vi "Message Based Application Example.vi"() -> ()   [LabVIEW 2014]
uses:
  <vilib>/Utility/error.llb/DialogType.ctl
  vilib/Message/Msg Post UI Message.vi
  vilib/Message/Msg Post Queue Message.vi
  vilib/Message/Msg Send Queue Message.vi
panel:
  in  "Button 2":bool
  in  "Button 1":bool
  in  "stop":bool
  # "Example buttons to create example events"
  # "Template for a Message Handling Framework-based VI. Add your controls (or menus or whatever) to the front panel here and edit the block diagram to complete the VI. You'll probably also want to delete this label!\n\nCopyright 2005 - 2016 Jason Sommerville\n\nPermision to use, modify and distribute this VI and its subVIs is granted under the BSD license."
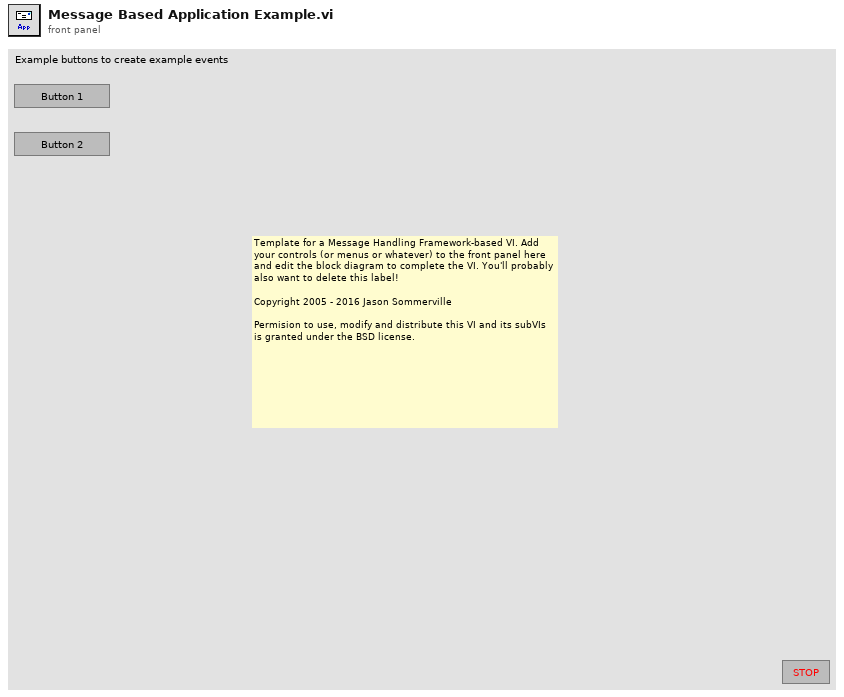
[diagram p1: front panel]
types:
  T1 = typedef "DialogType.ctl" = u16
  T2 = enum16{"Left Button", "Center Button", "Right Button", "Window Close"}
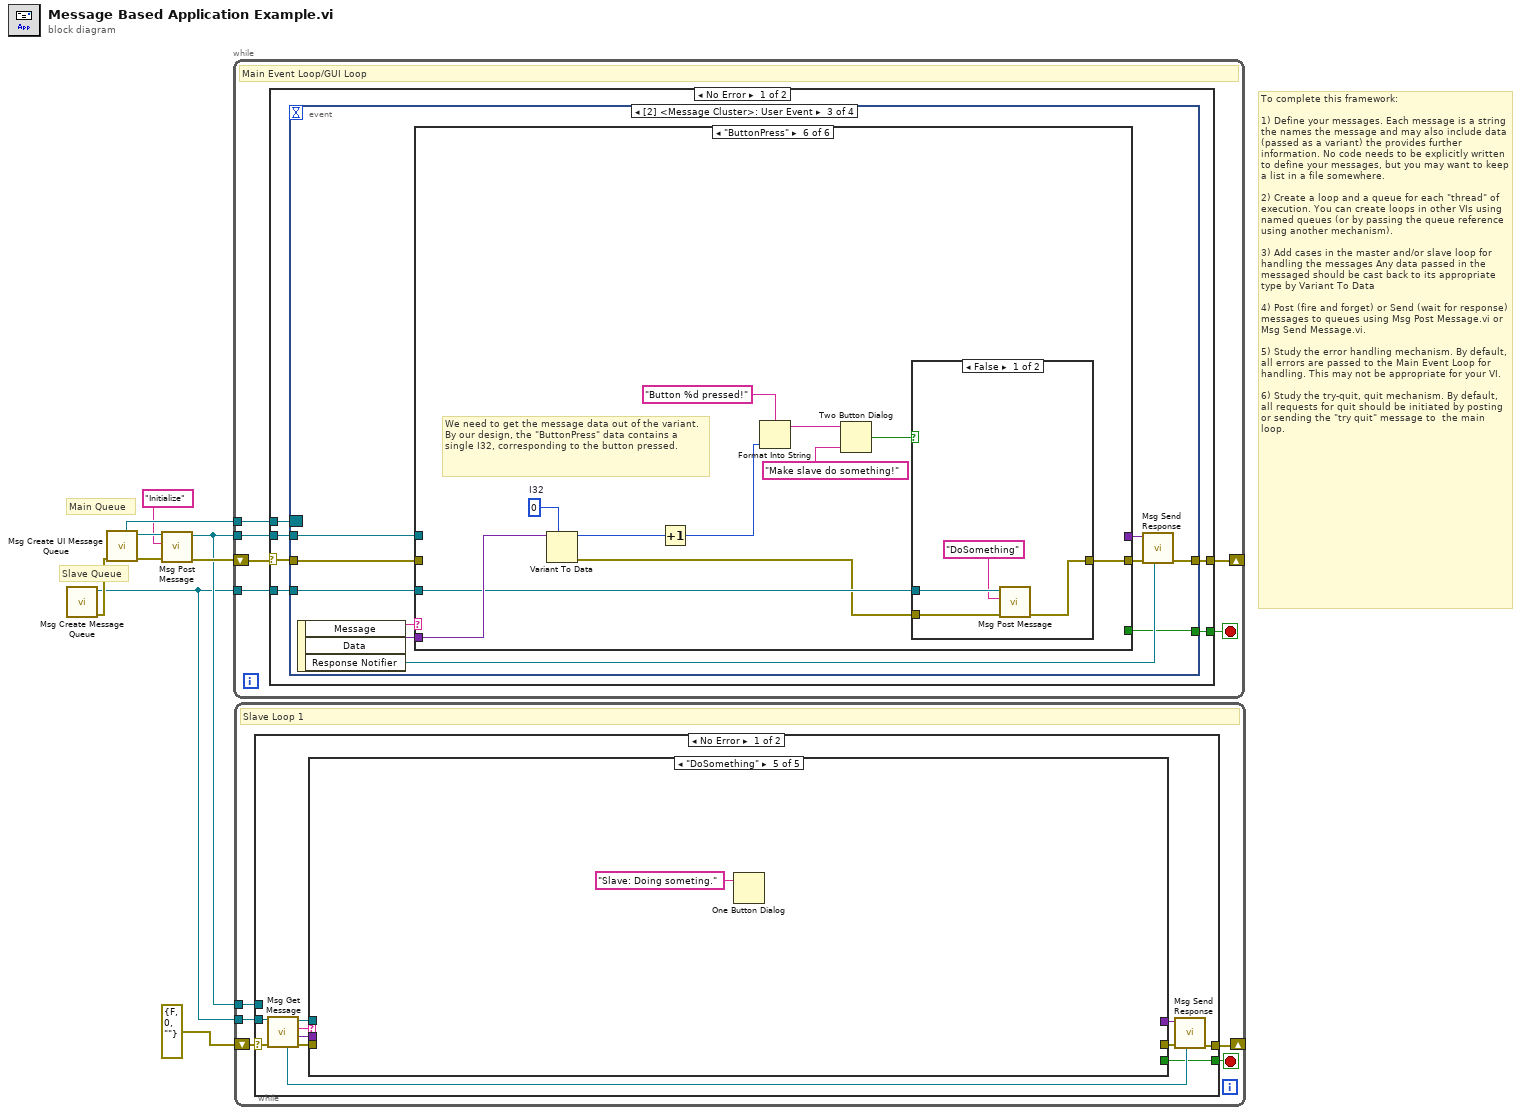
[diagram p0: block diagram]
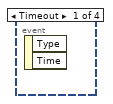
[diagram p2: hidden frame]
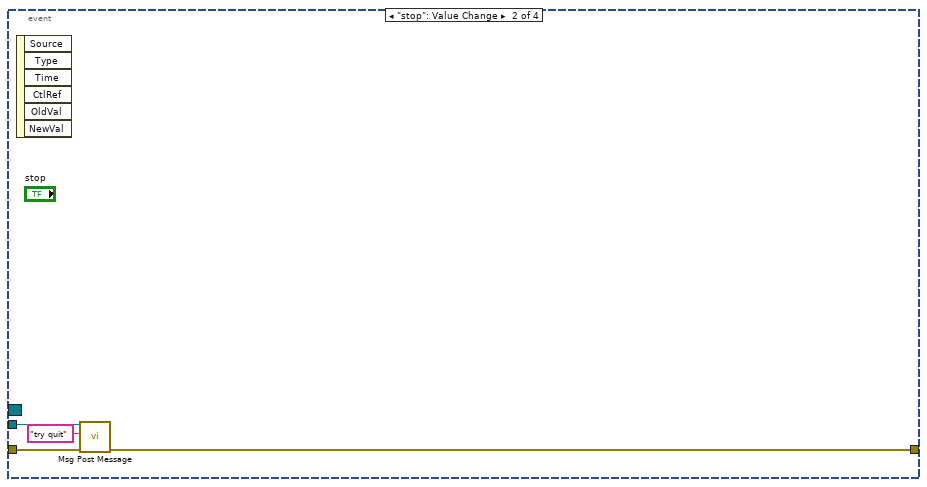
[diagram p3: hidden frame]
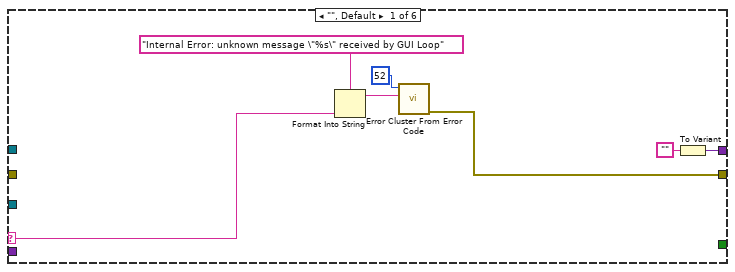
[diagram p4: hidden frame]
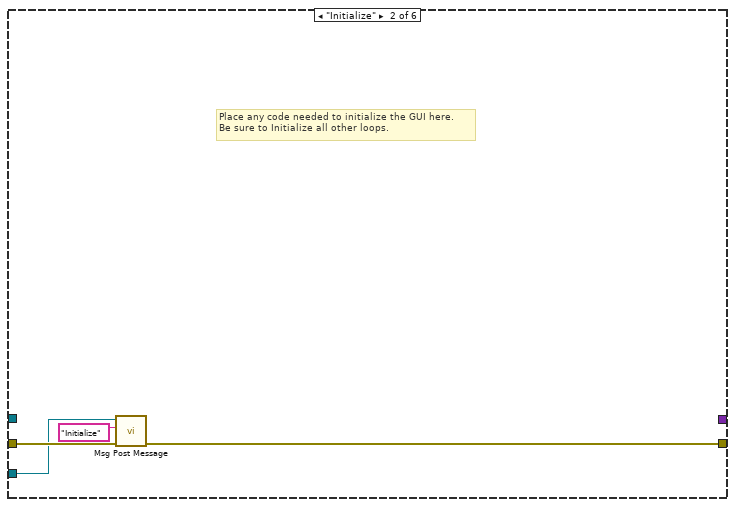
[diagram p5: hidden frame]
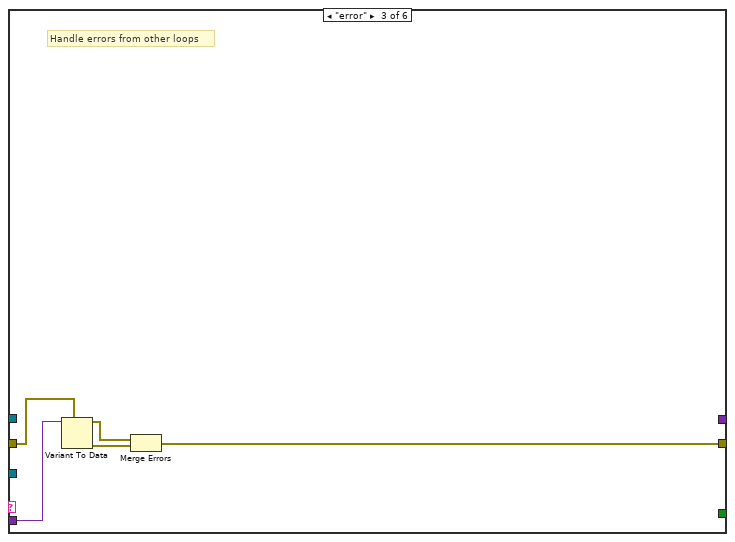
[diagram p6: hidden frame]
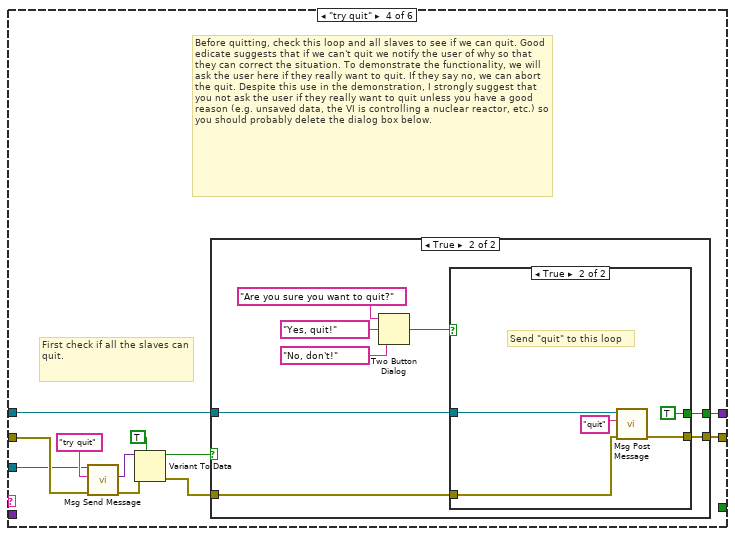
[diagram p7: hidden frame]
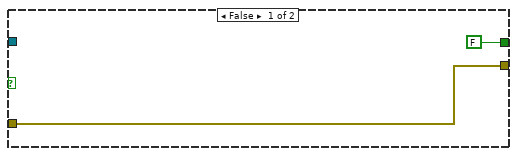
[diagram p8: hidden frame]
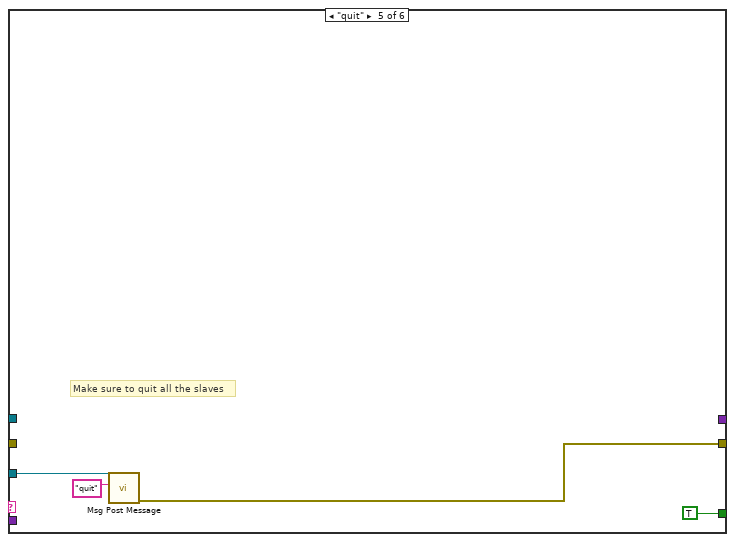
[diagram p10: hidden frame]
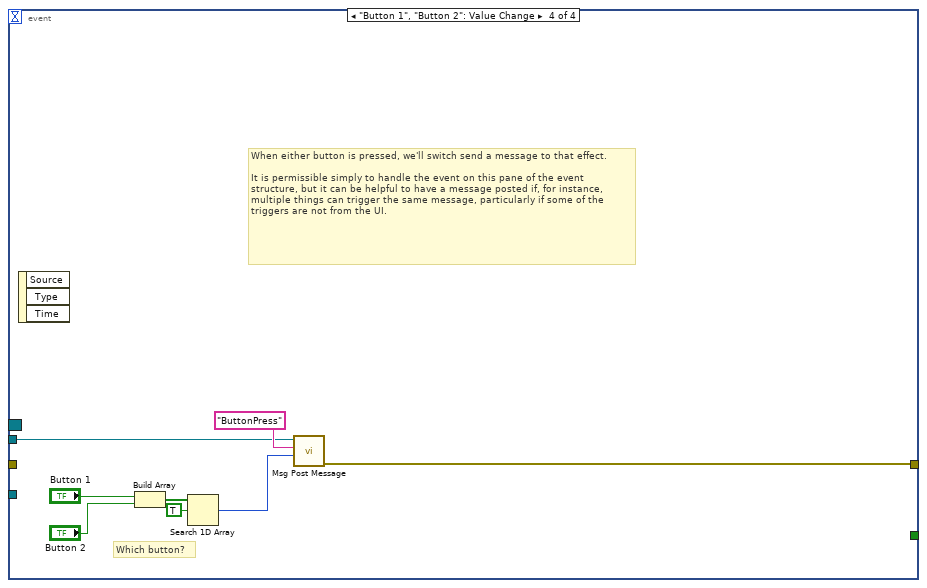
[diagram p12: hidden frame]
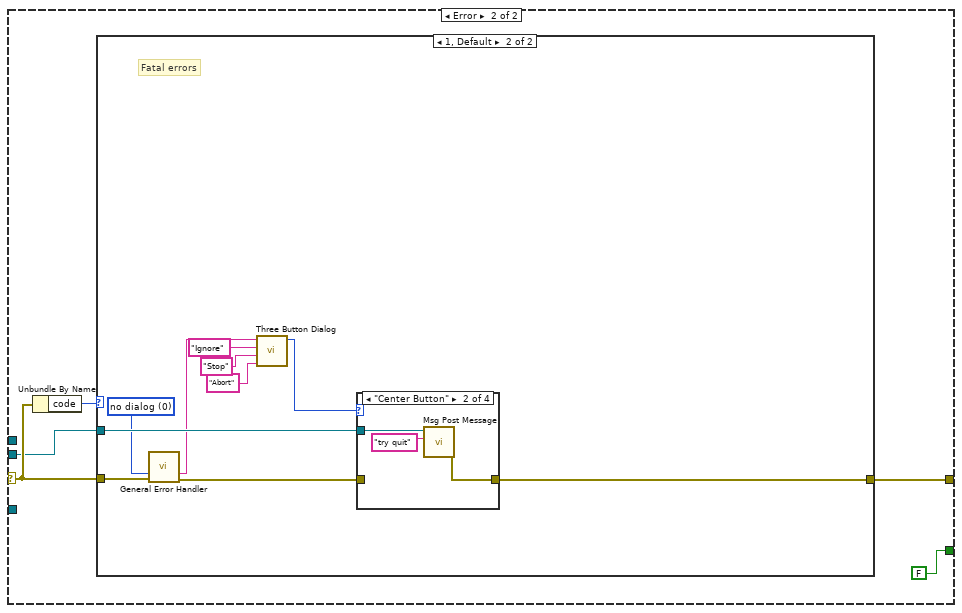
[diagram p13: hidden frame]
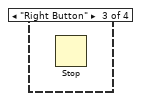
[diagram p16: hidden frame]
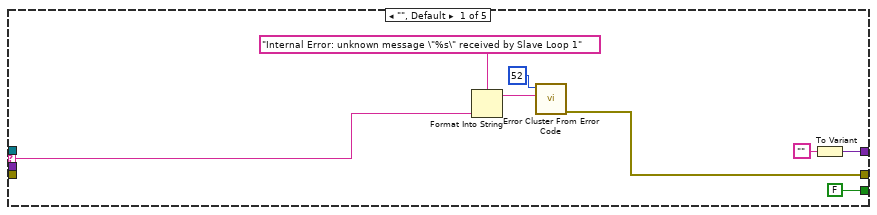
[diagram p18: hidden frame]
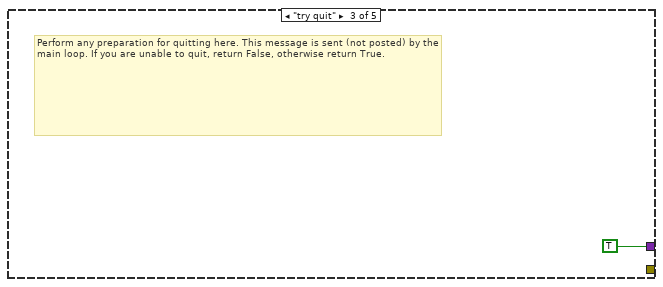
[diagram p20: hidden frame]
diagram:
  # "To complete this framework:\n\n1) Define your messages. Each message is a string the names the message and may also include data (passed as a variant) the provides further information. No code needs to be explicitly written to define your messages, but you may want to keep a list in a file somewhere.\n\n2) Create a loop and a queue for each \"thread\" of execution. You can create loops in other VIs using named queues (or by passing the queue reference using another mechanism).\n\n3) Add cases in the master and/or slave loop for handling the messages Any data passed in the messaged should be cast back to its appropriate type by Variant To Data\n\n4) Post (fire and forget) or Send (wait for response) messages to queues using Msg Post Message.vi or Msg Send Message.vi.\n\n5) Study the error handling mechanism. By default, all errors are passed to the Main Event Loop for handling. This may not be appropriate for your VI.\n\n6) Study the try-quit, quit mechanism. By default, all requests for quit should be initiated by posting or sending the \"try quit\" message to  the main loop."
  # "Main Queue"
  # "Slave Queue"
  n1 = call "Msg Create Message Queue.vi"() -> ("error out"=w5:errorcluster, "queue out"=w2:refnum<queue>)  [unwired: 7 in, 1 out]
  n2 = call "Msg Create UI Message Queue.vi"("error in (no error)"=w5) -> ("error out"=w6:errorcluster, "user event"=w8:refnum<user-event>, "Event Registration Refnum out"=w9:refnum<event-registration>)  [unwired: 6 in]
  n3 = call-poly "Msg Post Message.vi"("error in (no error)"=w6, "Message"="Initialize", "user event"=w8) -> ("error out"=w4:errorcluster, "user event out"=w3:refnum<user-event>)  [unwired: 4 in, 1 out]
  n4 = while {
    tunnel: w9 -> [w14]
    shift-right: [w12] -> _
    shift-left: w4 -> [w10]
    tunnel: w3 -> [w13]
    tunnel: w2 -> [w11]
    stop <- w15 stop-if-true
    # "Main Event Loop/GUI Loop"
    n5 = case shown="No Error" w10 {
      selector: w10 -> [w16 w109]
      tunnel: [w21 FALSE] -> w15
      tunnel: w14 -> [w20 _]
      tunnel: w13 -> [w19 w108]
      tunnel: [w18 w107] -> w12
      tunnel: w11 -> [w17 _]
      frame No Error {
        n6 = event shown="[2] <Message Cluster>: User Event" {
          selector: w20 -> [_ _ _ _]
          dyn-events: _ -> [_ _ _ _]
          timeout: _ -> [_ _ _ _]
          tunnel: [_ _ w26 _] -> w21
          tunnel: w19 -> [_ w25 w27 w105]
          tunnel: w16 -> [_ w24 w32 _]
          tunnel: [_ w23 w30 w99] -> w18
          tunnel: w17 -> [_ _ w28 _]
          event Timeout {
            n7 = event-data() -> ()  [unwired: 1 in, 2 out]
          }
          event "stop": Value Change {
            n8 = event-data() -> ()  [unwired: 1 in, 6 out]
            n9 = call-poly "Msg Post Message.vi"("error in (no error)"=w24, "Message"="try quit", "user event"=w25) -> ("error out"=w23:errorcluster)  [unwired: 4 in, 2 out]
          }
          event User Event {
            n10 = event-data() -> ("Message"=w35:string, "Data"=w29:variant, "Response Notifier"=w33:refnum<notifier>)  [unwired: 1 in]
            n11 = case shown="\"ButtonPress\"" w35 {
              selector: w35 -> [w40 _ _ _ _ _]
              tunnel: [w41 _ _ w55 _ _] -> w34
              tunnel: w32 -> [_ w46 w50 w62 _ _]
              tunnel: [w36 w43 w47 w56 w79 w84] -> w31
              tunnel: w29 -> [_ _ w51 _ _ w93]
              tunnel: w28 -> [_ w45 _ w53 w80 w86]
              tunnel: w27 -> [_ _ _ w57 _ _]
              tunnel: [_ _ _ _ TRUE _] -> w26
              frame "", Default {
                n12 = Format Into String(format string="Internal Error: unknown message \"%s\" received by GUI Loop" ("error message (\"\")"), w40) -> (resulting string=w37:string)  [unwired: 2 in, 1 out]
                n13 = call <vilib>:"Error Cluster From Error Code.vi"("error message (\"\")"=w37, "error code (0)"=52) -> ("error out"=w36:errorcluster)  [unwired: 7 in]
                n14 = To Variant(anything="") -> (Variant=w41:variant)
              }
              frame "Initialize" {
                # "Place any code needed to initialize the GUI here. \nBe sure to Initialize all other loops."
                n15 = call-poly "Msg Post Message.vi"("error in (no error)"=w46, "Message"="Initialize", "queue"=w45) -> ("error out"=w43:errorcluster)  [unwired: 4 in, 2 out]
              }
              frame "error" {
                # "Handle errors from other loops"
                n16 = Variant To Data(type=w50, Variant=w51) -> (data=w49:errorcluster, error out=w48:errorcluster)  [unwired: 1 in]
                n17 = Merge Errors(w49, w48) -> (w47:errorcluster)
              }
              frame "try quit" {
                # "Before quitting, check this loop and all slaves to see if we can quit. Good edicate suggests that if we can't quit we notify the user of why so that they can correct the situation. To demonstrate the functionality, we will ask the user here if they really want to quit. If they say no, we can abort the quit. Despite this use in the demonstration, I strongly suggest that you not ask the user if they really want to quit unless you have a good reason (e.g. unsaved data, the VI is controlling a nuclear reactor, etc.) so you should probably delete the dialog box below."
                # "First check if all the slaves can quit."
                n18 = call-poly "Msg Send Message.vi"("error in (no error)"=w62, "Message"="try quit", "queue"=w53) -> ("error out"=w60:errorcluster, "response"=w54:variant)  [unwired: 3 in, 2 out]
                n19 = Variant To Data(error in=w60, type=TRUE, Variant=w54) -> (data=w52:bool, error out=w58:errorcluster)
                n20 = case shown="True" w52 {
                  tunnel: w58 -> [w64 w71]
                  tunnel: w57 -> [_ w72]
                  tunnel: [w64 w70] -> w56
                  tunnel: [FALSE w69] -> w55
                  frame False {
                  }
                  frame True {
                    n21 = Two Button Dialog(message="Are you sure you want to quit?", 1:"No, don't!" ("T button name (\"OK\")"), 2:"Yes, quit!" ("T button name (\"OK\")")) -> (T button?=w65:bool)
                    n22 = case shown="True" w65 {
                      tunnel: w72 -> [_ w78]
                      tunnel: w71 -> [w73 w76]
                      tunnel: [w73 w75] -> w70
                      tunnel: [_ TRUE] -> w69
                      frame False {
                      }
                      frame True {
                        # "Send \"quit\" to this loop"
                        n23 = call-poly "Msg Post Message.vi"("error in (no error)"=w76, "Message"="quit", "user event"=w78) -> ("error out"=w75:errorcluster)  [unwired: 4 in, 2 out]
                      }
                    }
                  }
                }
              }
              frame "quit" {
                # "Make sure to quit all the slaves"
                n24 = call-poly "Msg Post Message.vi"("Message"="quit", "queue"=w80) -> ("error out"=w79:errorcluster)  [unwired: 5 in, 2 out]
              }
              frame "ButtonPress" {
                w92 = 0  # I32
                # "We need to get the message data out of the variant. By our design, the \"ButtonPress\" data contains a single I32, corresponding to the button pressed."
                n25 = Variant To Data(type=w92, Variant=w93) -> (data=w91:i32, error out=w85:errorcluster)  [unwired: 1 in]
                n26 = Increment(x=w91) -> (x+1=w83:i32)
                n27 = Format Into String(format string="Button %d pressed!", w83) -> (resulting string=w89:string)  [unwired: 2 in, 1 out]
                n28 = Two Button Dialog(message=w89, 1:"Make slave do something!" ("F button name (\"Cancel\")")) -> (T button?=w87:bool)  [unwired: 1 in]
                n29 = case shown="False" w87 {
                  tunnel: w86 -> [w97 _]
                  tunnel: w85 -> [w95 w98]
                  tunnel: [w94 w98] -> w84
                  frame False {
                    n30 = call-poly "Msg Post Message.vi"("error in (no error)"=w95, "Message"="DoSomething", "queue"=w97) -> ("error out"=w94:errorcluster)  [unwired: 4 in, 2 out]
                  }
                  frame True {
                  }
                }
              }
            }
            n31 = call "Msg Send Response.vi"("Response Notifier"=w33, "error in (no error)"=w31, "response"=w34) -> ("error out"=w30:errorcluster)  [unwired: 6 in]
          }
          event "Button 1", "Button 2": Value Change {
            # "Which button?"
            # "When either button is pressed, we'll switch send a message to that effect.\n\nIt is permissible simply to handle the event on this pane of the event structure, but it can be helpful to have a message posted if, for instance, multiple things can trigger the same message, particularly if some of the triggers are not from the UI."
            n32 = event-data() -> ()  [unwired: 1 in, 3 out]
            n33 = Build Array("Button 1", "Button 2") -> (w102:bool[])
            n34 = Search 1D Array(1D array=w102, element=TRUE) -> (index of element=w100:i32)  [unwired: 1 in]
            n35 = call-poly "Msg Post Message.vi"("Data"=w100, "Message"="ButtonPress", "user event"=w105) -> ("error out"=w99:errorcluster)  [unwired: 4 in, 2 out]
          }
        }
      }
      frame Error {
        n36 = Unbundle By Name(w109) -> ("code"=w110:i32)
        n37 = case shown="1, Default" w110 {
          tunnel: w109 -> [_ w121]
          tunnel: w108 -> [_ w120]
          tunnel: [_ w118] -> w107
          frame 0 {
            # "Ignore these errors"
          }
          frame 1, Default {
            w117 = T1 0 items=["no dialog", "OK message", "continue or stop message", "OK message + warnings", "continue/stop + warnings"] ("type of dialog (OK msg:1)")
            # "Fatal errors"
            n38 = call <vilib>:"General Error Handler.vi"("type of dialog (OK msg:1)"=w117, "error in (no error)"=w121) -> ("message"=w116:string, "error out"=w119:errorcluster)  [unwired: 9 in, 3 out]
            n39 = call <vilib>:"Three Button Dialog.vi"("Right Button Text (\"Cancel\")"="Abort" ("Right Button Text (\"Cancel\")"), "Center Button Text (\"No\")"="Stop" ("Center Button Text (\"No\")"), "Left Button Text (\"Yes\")"="Ignore" ("Left Button Text (\"Yes\")"), "message"=w116) -> ("Which Button?"=w112:T2)  [unwired: 7 in]
            n40 = case shown="\"Center Button\"" w112 {
              tunnel: w120 -> [_ w124 _ _]
              tunnel: w119 -> [_ _ _ _]
              tunnel: [_ w122 _ _] -> w118
              frame "Left Button", Default {
              }
              frame "Center Button" {
                n41 = call-poly "Msg Post Message.vi"("Message"="try quit", "user event"=w124) -> ("error out"=w122:errorcluster)  [unwired: 5 in, 2 out]
              }
              frame "Right Button" {
                n42 = Stop() -> ()  [unwired: 1 in]
              }
              frame "Window Close" {
              }
            }
          }
        }
      }
    }
  }
  n43 = while {
    tunnel: w3 -> [w125]
    tunnel: w2 -> [w129]
    shift-right: [w128] -> _
    shift-left: errorcluster {"status"=FALSE, "code"=0, "source"=""} ("error out") -> [w126]
    stop <- w127 stop-if-true
    # "Slave Loop 1"
    n44 = case shown="No Error" w126 {
      selector: w126 -> [w130 w153]
      tunnel: w129 -> [w140 _]
      tunnel: [w134 w152] -> w128
      tunnel: [w131 _] -> w127
      tunnel: w125 -> [_ w155]
      frame No Error {
        n45 = call "Msg Get Message.vi"("queue"=w140, "error in (no error)"=w130) -> ("Response Notifier"=w133:refnum<notifier>, "queue out"=w136:refnum<queue>, "Message"=w138:string, "Data"=w137:variant, "error out"=w139:errorcluster)  [unwired: 2 in]
        n46 = case shown="\"DoSomething\"" w138 {
          selector: w138 -> [w141 _ _ _ _]
          tunnel: [w142 _ _ _ _] -> w135
          tunnel: w139 -> [_ _ _ _ _]
          tunnel: w137 -> [_ _ _ _ _]
          tunnel: w136 -> [_ _ _ _ _]
          tunnel: [w147 _ TRUE _ _] -> w132
          tunnel: [FALSE _ _ TRUE _] -> w131
          frame "", Default {
            n47 = Format Into String(format string="Internal Error: unknown message \"%s\" received by Slave Loop 1" ("error message (\"\")"), w141) -> (resulting string=w145:string)  [unwired: 2 in, 1 out]
            n48 = call <vilib>:"Error Cluster From Error Code.vi"("error message (\"\")"=w145, "error code (0)"=52) -> ("error out"=w142:errorcluster)  [unwired: 7 in]
            n49 = To Variant(anything="") -> (Variant=w147:variant)
          }
          frame "Initialize" {
            # "Place any code needed to initialize the Slave Loop here."
          }
          frame "try quit" {
            # "Perform any preparation for quitting here. This message is sent (not posted) by the main loop. If you are unable to quit, return False, otherwise return True."
          }
          frame "quit" {
          }
          frame "DoSomething" {
            n50 = One Button Dialog(message="Slave: Doing someting.") -> ()  [unwired: 1 in, 1 out]
          }
        }
        n51 = call "Msg Send Response.vi"("Response Notifier"=w133, "error in (no error)"=w135, "response"=w132) -> ("error out"=w134:errorcluster)  [unwired: 6 in]
      }
      frame Error {
        # "By default, send errors to the main loop for handling."
        n52 = call-poly "Msg Post Message.vi"("Data"=w153, "Message"="error", "user event"=w155) -> ("error out"=w152:errorcluster)  [unwired: 4 in, 2 out]
      }
    }
  }
